vi "Untitled 2.vi"() -> ()   [LabVIEW 2019]
uses:
  <vilib>/Utility/file.llb/Read Delimited Spreadsheet (DBL).vi
  <vilib>/Analysis/NI_AALBase.lvlib
panel:
  out "standard deviation":dbl format="%0.2f"
  out "mean":dbl format="%0.2f"
  in  "file path (dialog if empty)":path=path "C:/Users/a0230251/Desktop/New Text Document.txt"
  out "Waveform Graph":dbl[](graph)
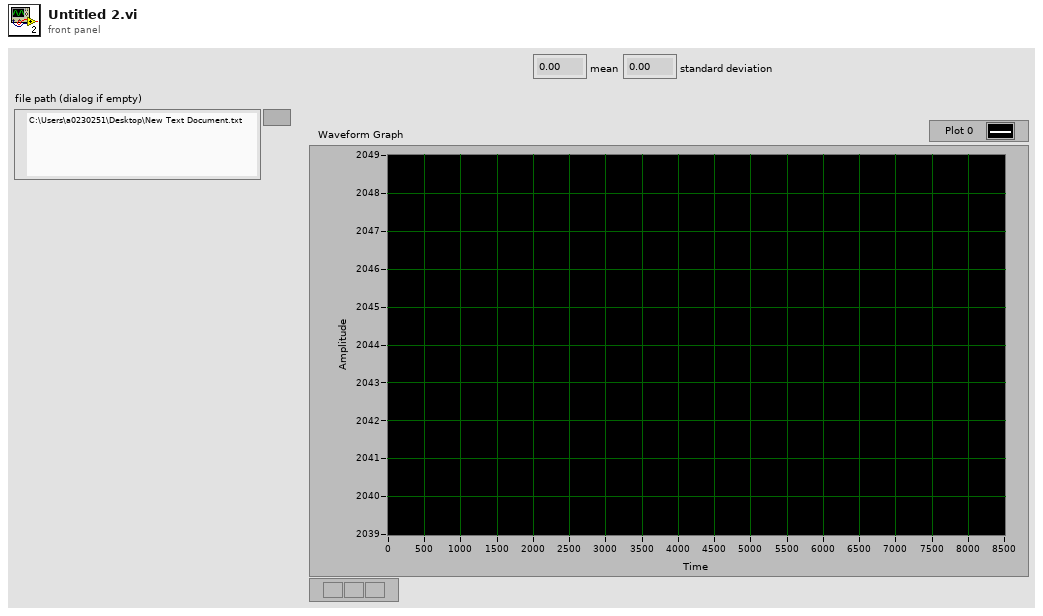
[diagram p1: front panel]
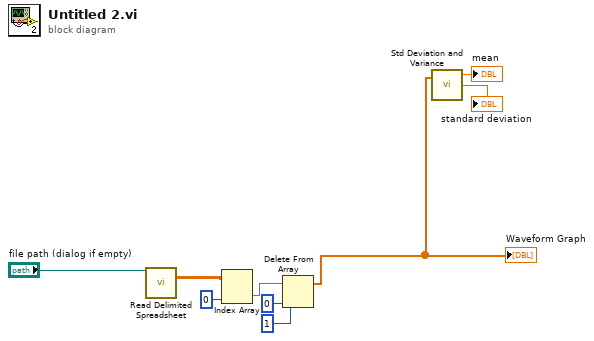
[diagram p0: block diagram]
diagram:
  n1 = call-poly <vilib>:"Read Delimited Spreadsheet.vi"("file path (dialog if empty)"="file path (dialog if empty)") -> ("all rows"=w6:dbl[][])  [unwired: 9 in, 5 out]
  n2 = Index Array(array=w6, index (col)=0 ("disabled index (col)")) -> (element=w4:dbl[])  [unwired: 1 in]
  n3 = Delete From Array(array=w4, length=1, index=0) -> (array with subset deleted=w3:dbl[])  [unwired: 1 out]
  "Waveform Graph" <- w3
  n4 = call <vilib>:"Std Deviation and Variance.vi"("X"=w3) -> ("mean"=→"mean":dbl, "standard deviation"=→"standard deviation":dbl)  [unwired: 1 in, 1 out]
